vi "Us1.vi"() -> ()   [LabVIEW 2021]
panel:
  out "Us1":dbl
  in  "k":dbl
  in  "z":dbl
  out "error out":errorcluster
  in  "error in (no error)":errorcluster
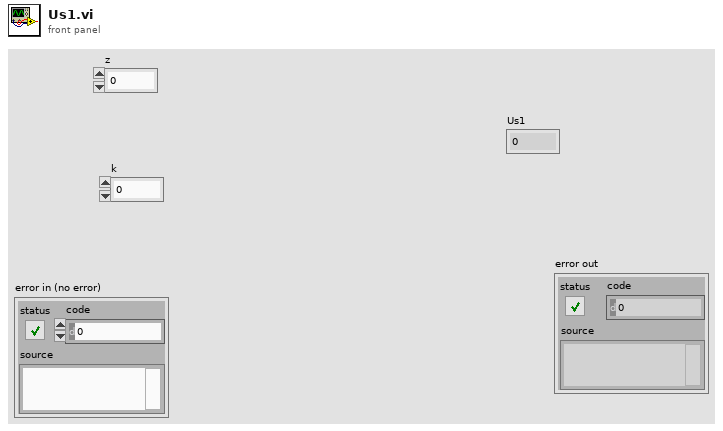
[diagram p1: front panel]
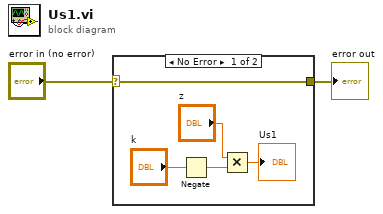
[diagram p0: block diagram]
diagram:
  n1 = case shown="No Error" "error in (no error)" {
    selector: "error in (no error)" -> [w3 w8]
    tunnel: [w3 w8] -> w1
    frame No Error {
      n2 = Negate(x="k") -> (-x=w6:dbl)
      n3 = Multiply(x="z", y=w6) -> (x*y=→"Us1":dbl)
    }
    frame Error {
    }
  }
  "error out" <- w1
